vi "获取雇员信息.vi"(8 "error in (no error)":errorcluster caption="错误输入（无错误）", 11 "雇员 输入":refnum<class "雇员.lvclass"> caption="DNL_LabVIEW Object in") -> (0 "error out":errorcluster caption="错误输出", 1 "年龄":u8, 2 "姓名":string, 3 "雇员 输出":refnum<class "雇员.lvclass"> caption="DNL_LabVIEW Object out", 4 "职务":string)   [LabVIEW 2011, in "迭代器.lvlib" / "雇员.lvclass"]
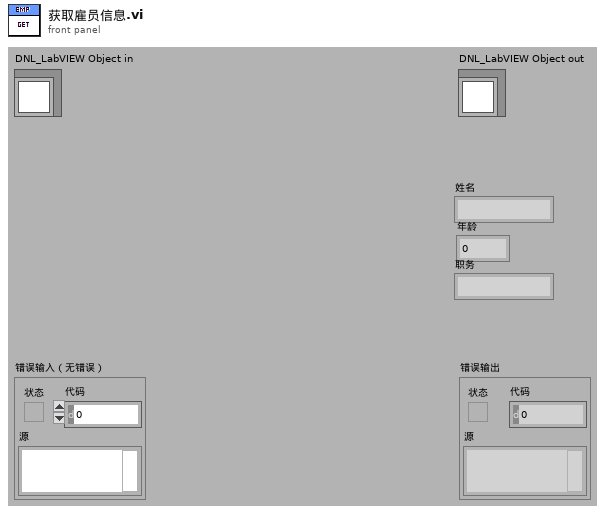
[diagram p1: front panel]
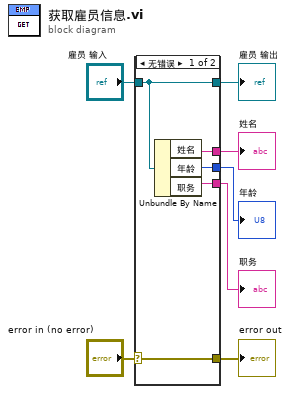
[diagram p0: block diagram]
diagram:
  n1 = case shown="无错误" "error in (no error)" {
    selector: "error in (no error)" -> [w12 w14]
    tunnel: [w12 w14] -> w6
    tunnel: [w11 w13] -> w4
    tunnel: "雇员 输入" -> [w11 w13]
    tunnel: [w10 _] -> w3
    tunnel: [w9 _] -> w2
    tunnel: [w8 _] -> w1
    frame No Error {
      n2 = Unbundle By Name(w11) -> ("姓名"=w10:string, "年龄"=w9:u8, "职务"=w8:string)
    }
    frame Error {
    }
  }
  "error out" <- w6
  "雇员 输出" <- w4
  "姓名" <- w3
  "年龄" <- w2
  "职务" <- w1
